vi "Stop Core.vi"(10 "final error code":i32, 11 "Timing Engine Tester in":refnum<class "Timing Engine Tester.lvclass">) -> (3 "Timing Engine Tester out":refnum<class "Timing Engine Tester.lvclass">)   [LabVIEW 2016, in "Assert API Components.lvlib" / "Assert Display.lvlib" / "Timing Engine Tester.lvlib" / "Timing Engine Tester.lvclass"]
doc: "(<B>Filename</B>: Actor Framework.lvlib:Actor.lvclass:Stop Core.vi)\n\nDefines what the actor does before it stops. Use the <B>final error code</B> input to determine whether the actor shut down in response to an error.\n\nBy default, this method does nothing. A descendant class may override it to define behavior, such as shutting down any processes the actor initiated in its override of the Actor Core method."
uses:
  Timing Engine Tester.lvclass
  Timing Engine Tester.lvclass/Timing Engine Tester.ctl
  <vilib>/ActorFramework/Actor/Actor.lvclass
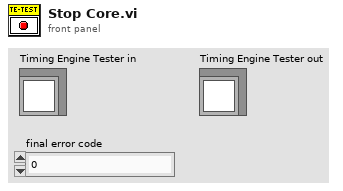
[diagram p1: front panel]
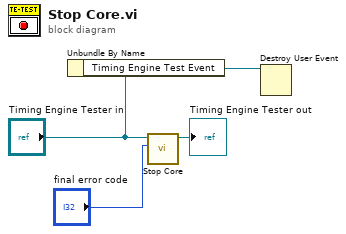
[diagram p0: block diagram]
diagram:
  n1 = Unbundle By Name("Timing Engine Tester in") -> ("Timing Engine Test Event"=w1:refnum<user-event>)
  n2 = call-parent "Stop Core.vi"("final error code"="final error code", "Actor in"="Timing Engine Tester in") -> ("Actor out"=→"Timing Engine Tester out":refnum<class "Timing Engine Tester.lvclass">)  [unwired: 9 in]
  n3 = Destroy User Event(user event=w1) -> ()  [unwired: 1 in, 1 out]
